vi "Generate Filename.vi"(9 "format  in":u16(ring) items=["TDMS", "CSV"], 11 "bustype in":string) -> (2 "filename":string)   [LabVIEW 2025, in "CAN-LIN Raw Bus Capture UI.lvlib"]
uses:
  CAN-LIN Raw Bus Capture UI.lvlib
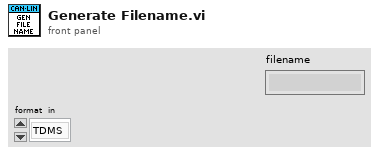
[diagram p1: front panel]
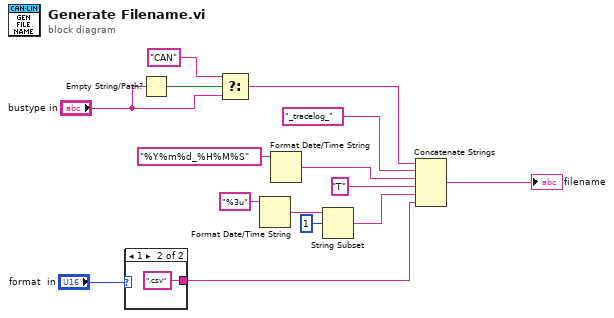
[diagram p0: block diagram]
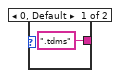
[diagram p2: hidden frame]
diagram:
  n1 = case shown="1" "format  in" {
    tunnel: [".tdms" ("search string/char (-)") ".csv" ("search string/char (-)")] -> w6
    frame 0, Default {
    }
    frame 1 {
    }
  }
  n2 = Empty String/Path?(string/path="bustype in") -> (empty?=w4:bool)
  n3 = Select(t="CAN", s=w4, f="bustype in") -> (s? t:f=w1:string)
  n4 = Format Date/Time String(time format string (%c)="%3u") -> (date/time string=w13:string)  [unwired: 2 in]
  n5 = Format Date/Time String(time format string (%c)="%Y%m%d_%H%M%S") -> (date/time string=w14:string)  [unwired: 2 in]
  n6 = String Subset(string=w13, offset (0)=1) -> (substring=w15:string)  [unwired: 1 in]
  n7 = Concatenate Strings(w1, "_tracelog_" ("string"), w14, "T" ("string"), w15, w6) -> (→"filename":string)
